vi "SettleDrift_v3.vi"() -> ()   [LabVIEW 2014]
uses:
  shared/CorrelImages (SubVI)Single.vi
  <userlib>/Nanonis Prog Interface V5/Nanonis Prog Interface.lvlib
panel:
  out "Saturation status":T1
  out "Compensation speeds (m/s)":cluster{"Vx":sgl, "Vy":sgl, "Vz":sgl} {"Vz" format="%#_5p"; "Vy" format="%#_5p"; "Vx" format="%#_5p"}
  out "Compensation status":bool
  in  "active drift compensation":bool
  out "y drift/sec":sgl format="%#_6p"
  out "x drift/sec":sgl format="%#_6p"
  out "seconds per image":dbl
  out "loops":i32
  in  "stop":bool
  out "x drift":sgl format="%#_6p"
  out "y drift":sgl format="%#_6p"
  out "y Drift":sgl(graph)
  out "X Drift":sgl(graph)
  in  "Drift correction Pixels":i32=256
  in  "Img Current":sgl=1e-11 format="%#_6p"
  in  "Img Bias (V)":sgl=-0.002 format="%_2p"
  in  "Img Speed":sgl=1.5e-07 format="%#_6p"
  in  "Channel index (0-23)":u8(ring) items=["Current"=0, "Z (m)"=14]
  # "Turn continuous scan off\ndo not use june 2017!"
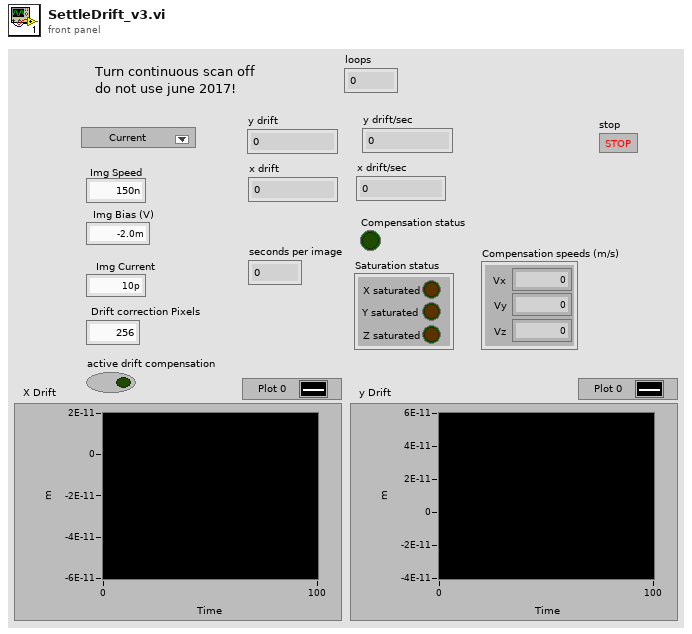
[diagram p1: front panel]
types:
  T1 = cluster{"X saturated":bool, "Y saturated":bool, "Z saturated":bool}
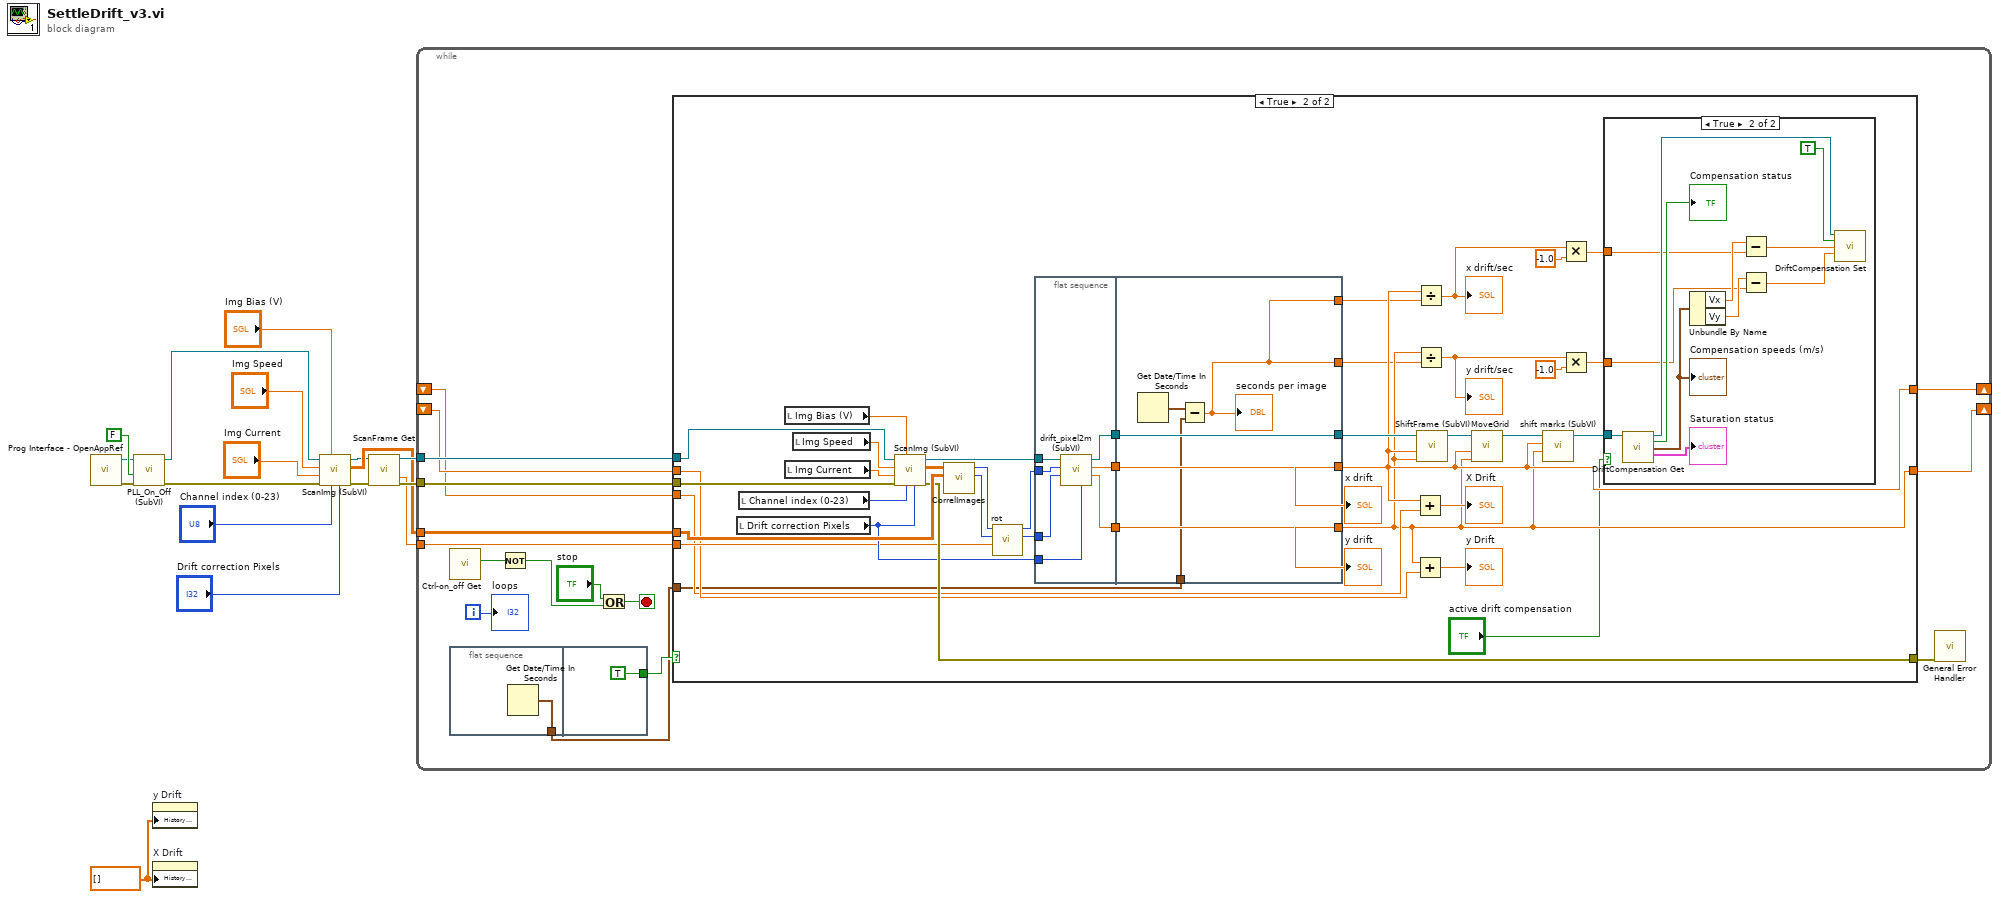
[diagram p0: block diagram]
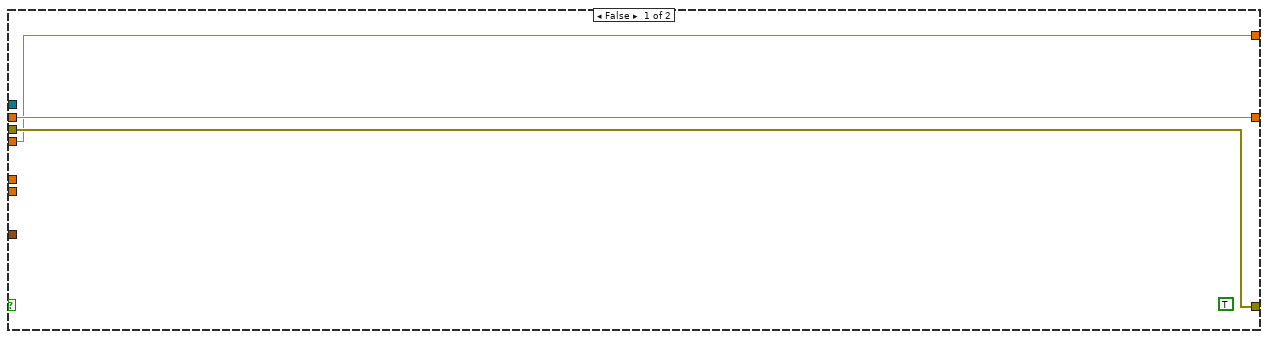
[diagram p2: hidden frame]
diagram:
  w1 = sgl[] [] ("History Data")
  n1 = call <userlib>:"Prog Interface - OpenAppRef.vi"() -> ("Error out"=w2:errorcluster, "Application reference"=w3:refnum<vi>)  [unwired: 6 in]
  n2 = call "PLL_On_Off (SubVI).vi"("error in (no error)"=w2, "Output ON/OFF (F=OFF)"=FALSE, "Application in"=w3) -> ("error out"=w8:errorcluster, "Application out"=w9:refnum<vi>)  [unwired: 7 in]
  n3 = property on="y Drift" class="WFChart (strict)"("History Data"=w1) -> ()  [unwired: 2 in, 2 out]
  n4 = property on="X Drift" class="WFChart (strict)"("History Data"=w1) -> ()  [unwired: 2 in, 2 out]
  n5 = call "ScanImg (SubVI).vi"("pixel"="Drift correction Pixels", "Channel index (0-23)"="Channel index (0-23)", "Bias (V)"="Img Bias (V)", "error in (no error)"=w8, "Current"="Img Current", "Img Speed"="Img Speed", "Application in"=w9) -> ("error out"=w4:errorcluster, "Img"=w15:dbl[][], "Application out"=w5:refnum<vi>)  [unwired: 2 in]
  n6 = call <userlib>:"ScanFrame Get.vi"("Application ref in"=w5, "error in (no error)"=w4) -> ("Application ref out"=w17:refnum<vi>, "Angle (deg)"=w14:sgl, "error out"=w16:errorcluster)  [unwired: 9 in, 2 out]
  n7 = while {
    tunnel: w17 -> [w33]
    tunnel: w16 -> [w32]
    tunnel: w15 -> [w31]
    tunnel: w14 -> [w30]
    shift-right: [w27] -> _
    shift-left: _ -> [w26]
    shift-right: [w28] -> _
    shift-left: _ -> [w25]
    i -> [w21]
    stop <- w24 stop-if-true
    n8 = call <userlib>:"Ctrl-on_off Get.vi"() -> ("Z-Controller on/off status"=w23:bool)  [unwired: 9 in, 2 out]
    n9 = flat-sequence {
      tunnel: [w34] -> w18
      tunnel: [TRUE] -> w19
      frame #0 {
        n10 = Get Date/Time In Seconds() -> (seconds since 1Jan1904=w34:timestamp)
      }
      frame #1 {
      }
    }
    n11 = Not(x=w23) -> (.not. x?=w22:bool)
    n12 = Or(x="stop", y=w22) -> (x .or. y?=w24:bool)
    n13 = case shown="True" w19 {
      tunnel: w31 -> [_ w77]
      tunnel: w33 -> [_ w61]
      tunnel: w32 -> [w38 w76]
      tunnel: [w38 w75] -> w20
      tunnel: w30 -> [_ w66]
      tunnel: [w36 w50] -> w28
      tunnel: [w37 w48] -> w27
      tunnel: w26 -> [w37 w56]
      tunnel: w25 -> [w36 w55]
      tunnel: w18 -> [_ w51]
      frame False {
        (unwired) TRUE ("DC active")
      }
      frame True {
        n14 = local read "Drift correction Pixels"() -> (w67:i32)
        n15 = local read "Channel index (0-23)"() -> (w70:u8)
        n16 = local read "Img Bias (V)"() -> (w71:sgl)
        n17 = local read "Img Current"() -> (w72:sgl)
        n18 = local read "Img Speed"() -> (w73:sgl)
        n19 = call "ScanImg (SubVI).vi"("pixel"=w67, "Channel index (0-23)"=w70, "Bias (V)"=w71, "error in (no error)"=w76, "Current"=w72, "Img Speed"=w73, "Application in"=w61) -> ("error out"=w75:errorcluster, "Img"=w74:dbl[][], "Application out"=w68:refnum<vi>)  [unwired: 2 in]
        n20 = call-poly "CorrelImages.vi"("Ref Array"=w77, "New Image"=w74) -> ("Y drift"=w63:i32, "X drift"=w65:i32)  [unwired: 6 in, 2 out]
        n21 = call "rot.vi"("angle"=w66, "y"=w63, "x"=w65) -> ("y'"=w62:i32, "x'"=w64:i32)  [unwired: 7 in]
        n22 = flat-sequence {
          tunnel: w68 -> [w95]
          tunnel: w67 -> [w94]
          tunnel: w64 -> [w93]
          tunnel: w62 -> [w92]
          tunnel: [w96] -> w54
          tunnel: [w91] -> w53
          tunnel: [w90] -> w52
          tunnel: [w100] -> w48
          tunnel: [w101] -> w50
          tunnel: [w102] -> w69
          tunnel: w54 -> [w102]
          tunnel: w53 -> [w101]
          tunnel: w52 -> [w100]
          tunnel: w51 -> [w98]
          tunnel: [w97] -> w49
          tunnel: [w97] -> w47
          frame #0 {
            n23 = call "drift_pixel2m (SubVI).vi"("Application in"=w95, "X drift"=w93, "Y drift"=w92, "Drift correction Pixels"=w94) -> ("Application out"=w96:refnum<vi>, "x drift"=w91:sgl, "y drift"=w90:sgl)  [unwired: 2 in, 1 out]
          }
          frame #1 {
            n24 = Get Date/Time In Seconds() -> (seconds since 1Jan1904=w99:timestamp)
            n25 = Subtract(x=w99, y=w98) -> (x-y=w97:dbl)
            "seconds per image" <- w97
          }
        }
        n26 = Add(x=w50, y=w55) -> (x+y=→"X Drift":sgl)
        n27 = Add(x=w48, y=w56) -> (x+y=→"y Drift":sgl)
        n28 = Divide(x=w50, y=w49) -> (x/y=w43:dbl)
        "x drift/sec" <- w43
        n29 = Divide(x=w48, y=w47) -> (x/y=w44:dbl)
        "y drift/sec" <- w44
        n30 = call "ShiftFrame (SubVI).vi"("Y shift"=w48, "X shift"=w50, "Application in"=w69) -> ("Application out"=w60:refnum<vi>)  [unwired: 8 in]
        n31 = call "MoveGrid.vi"("y"=w48, "x"=w50, "Application ref in"=w60) -> ("Application ref out"=w59:refnum<vi>)  [unwired: 7 in, 1 out]
        n32 = call "shift marks (SubVI).vi"("y"=w48, "x"=w50, "Application in"=w59) -> ("Application out"=w45:refnum<vi>)  [unwired: 7 in, 1 out]
        n33 = Multiply(x=w43, y=-1.0) -> (x*y=w41:dbl)
        n34 = Multiply(x=w44, y=-1.0) -> (x*y=w42:dbl)
        n35 = case shown="True" "active drift compensation" {
          tunnel: w45 -> [_ w89]
          tunnel: w42 -> [_ w81]
          tunnel: w41 -> [_ w80]
          frame False {
          }
          frame True {
            n36 = call <userlib>:"DriftCompensation Get.vi"("Application ref in"=w89) -> ("Application ref out"=w88:refnum<vi>, "Compensation status"=→"Compensation status":bool, "Compensation speeds (m/s)"=w84:cluster{"Vx":sgl, "Vy":sgl, "Vz":sgl}, "Saturation status"=→"Saturation status":T1)  [unwired: 10 in, 1 out]
            "Compensation speeds (m/s)" <- w84
            n37 = Unbundle By Name(w84) -> ("Vx"=w83:sgl, "Vy"=w82:sgl)
            n38 = Subtract(x=w83, y=w80) -> (x-y=w79:dbl)
            n39 = Subtract(x=w82, y=w81) -> (x-y=w78:dbl)
            n40 = call <userlib>:"DriftCompensation Set.vi"("Application ref in"=w88, "Compensation On/Off"=TRUE, "Vx (m/s)"=w79, "Vy (m/s)"=w78) -> ()  [unwired: 10 in, 2 out]
          }
        }
        "y drift" <- w48
        "x drift" <- w50
      }
    }
    n41 = call <vilib>:"General Error Handler.vi"("error in (no error)"=w20) -> ()  [unwired: 10 in, 5 out]
    "loops" <- w21
  }
